vi "TmeDomain_TimeControl_Play_Pause.vi"() -> ()   [LabVIEW 2020]
uses:
  <vilib>/Waveform/WDTOps.llb/WDT Index Channel DBL.vi
panel:
  out "Pause Iterations":i32
  in  "Enum":enum16{"Pause", "Play"}(ring)=enum."Play"
  out "Paused Final Graph":dbl[][](graph)
  out "Raw waveform":dbl(graph)
  out "Iteration":i32
  out "Actual waveform":dbl(graph)
  in  "Sampling Time (s)":dbl step=0.1
  out "Sampled index":dbl
  out "Time elapsed (s)":dbl
  out "Time Elapsed (min)":dbl
  in  "?":bool
  out "Final Graph":dbl[](graph)
  out "dt":dbl
  in  "File origin":path
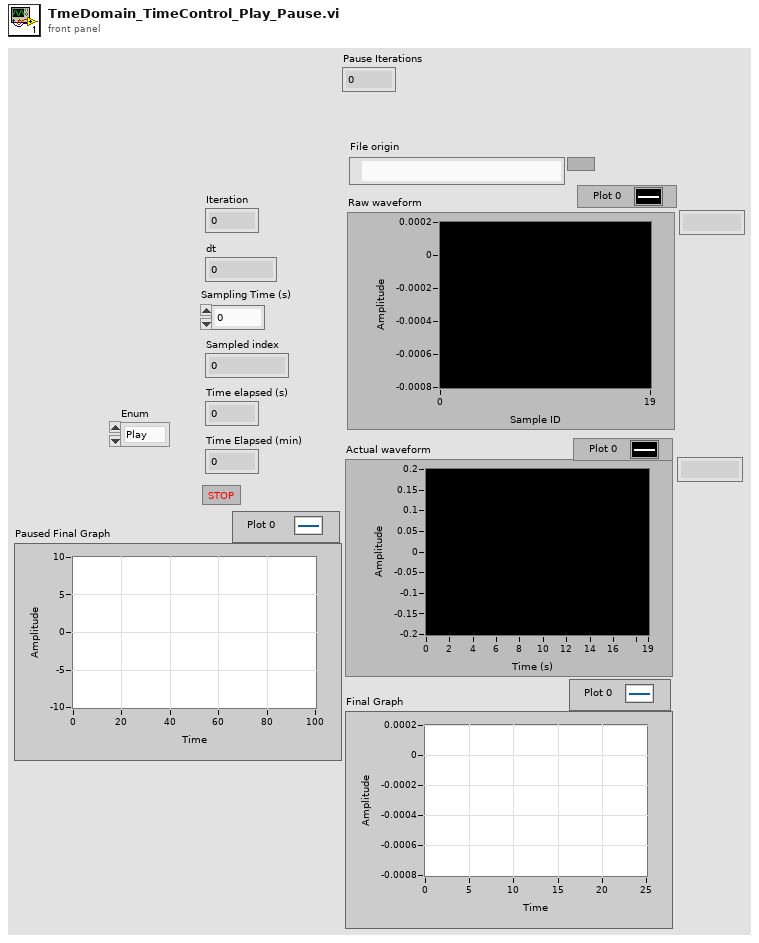
[diagram p1: front panel]
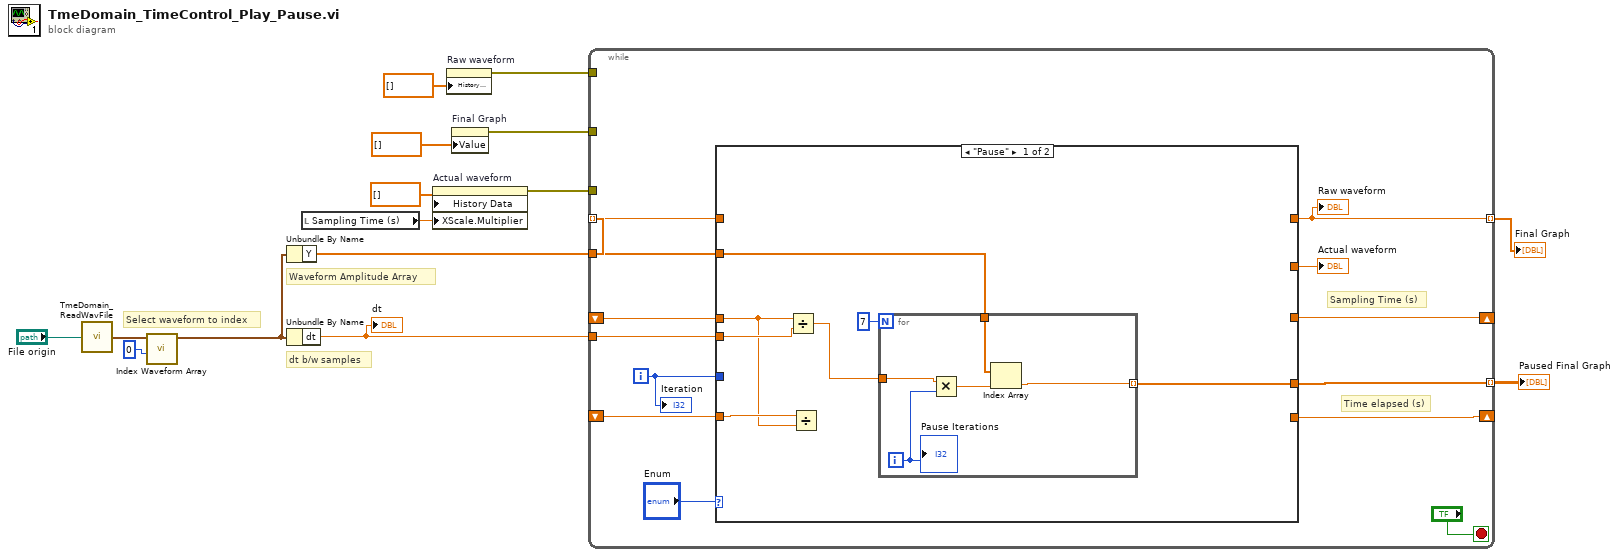
[diagram p0: block diagram]
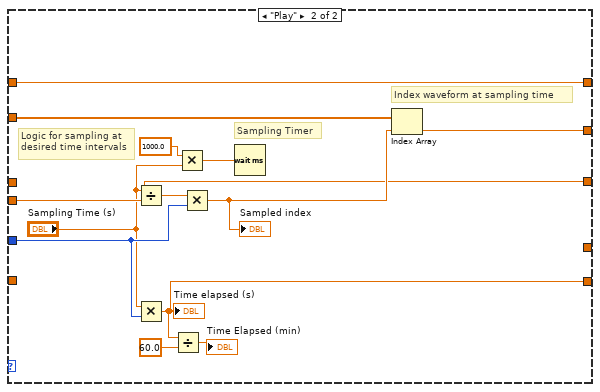
[diagram p2: hidden frame]
diagram:
  # "dt b/w samples"
  # "Waveform Amplitude Array"
  # "Select waveform to index"
  n1 = call "TmeDomain_ReadWavFile.vi"("path"="File origin") -> ("data"=w14:waveform(dbl)[])
  n2 = call-poly <vilib>:"Index Waveform Array.vi"("index"=0, "waveform array"=w14) -> ("waveform"=w12:waveform(dbl))  [unwired: 8 in, 1 out]
  n3 = Unbundle By Name(w12) -> ("Y"=w11:dbl[])
  n4 = Unbundle By Name(w12) -> ("dt"=w10:dbl)
  "dt" <- w10
  n5 = local read "Sampling Time (s)"() -> (w2:dbl)
  n6 = property on="Actual waveform" class="WFChart (strict)"("History Data"=dbl[] [], "XScale.Multiplier"=w2) -> (error out=w8:errorcluster)  [unwired: 2 in, 1 out]
  n7 = property on="Raw waveform" class="WFChart (strict)"("History Data"=dbl[] []) -> (error out=w5:errorcluster)  [unwired: 2 in, 1 out]
  n8 = property on="Final Graph" class="WFGraph (strict)"("Value"=dbl[] [] ("Final Graph")) -> (error out=w4:errorcluster)  [unwired: 2 in, 1 out]
  n9 = while {
    tunnel: w11 -> [w23] mode=indexing
    tunnel: w11 -> [w28]
    tunnel: w10 -> [w26]
    tunnel: [w22] -> w9 mode=indexing
    tunnel: w8 -> [_]
    tunnel: w5 -> [_]
    tunnel: w4 -> [_]
    shift-right: [w21] -> _
    shift-left: _ -> [w20]
    shift-right: [w19] -> _
    shift-left: _ -> [w18]
    tunnel: [w17] -> w1 mode=indexing
    i -> [w25]
    stop <- "?" stop-if-true
    # "Time elapsed (s)"
    # "Sampling Time (s)"
    n10 = case shown="\"Pause\"" "Enum" {
      tunnel: w28 -> [w31 w53]
      tunnel: [_ w52] -> w27
      tunnel: w26 -> [w35 w51]
      tunnel: w25 -> [_ w46]
      tunnel: w23 -> [_ w43]
      tunnel: [_ w43] -> w22
      tunnel: [_ "Sampling Time (s)"] -> w21
      tunnel: w20 -> [w33 _]
      tunnel: [_ w41] -> w19
      tunnel: w18 -> [w34 _]
      tunnel: [w30 _] -> w17
      frame "Pause" {
        n11 = Divide(x=w33, y=w35) -> (x/y=w32:dbl)
        n12 = Divide(x=w34, y=w33) -> ()  [unwired: 1 out]
        n13 = for {
          N: 7 -> [_]
          tunnel: w32 -> [w39]
          tunnel: w31 -> [w37]
          tunnel: [w36] -> w30 mode=indexing
          i -> [w40]
          n14 = Multiply(x=w39, y=w40) -> (x*y=w38:dbl)
          n15 = Index Array(array=w37, index=w38) -> (element=w36:dbl)
          "Pause Iterations" <- w40
        }
      }
      frame "Play" {
        # "Logic for sampling at\ndesired time intervals"
        # "Index waveform at sampling time"
        # "Sampling Timer"
        n16 = Divide(x="Sampling Time (s)", y=w51) -> (x/y=w48:dbl)
        n17 = Multiply(x="Sampling Time (s)", y=w46) -> (x*y=w41:dbl)
        "Time elapsed (s)" <- w41
        n18 = Divide(x=w41, y=60.0) -> (x/y=→"Time Elapsed (min)":dbl)
        n19 = Multiply(x=1000.0, y="Sampling Time (s)") -> (x*y=w49:dbl)
        n20 = Multiply(x=w48, y=w46) -> (x*y=w47:dbl)
        "Sampled index" <- w47
        n21 = Wait (ms)(milliseconds to wait=w49) -> ()  [unwired: 1 out]
        n22 = Index Array(array=w53, index=w47) -> (element=w52:dbl)
      }
    }
    "Raw waveform" <- w22
    "Actual waveform" <- w27
    "Iteration" <- w25
  }
  "Final Graph" <- w9
  "Paused Final Graph" <- w1
